vi "Write eLogLvl.vi"(8 "error in (no error)":errorcluster, 10 "eLogLvl":T1, 11 "Config in":refnum<class "Config.lvclass">) -> (0 "error out":errorcluster, 3 "Config out":refnum<class "Config.lvclass">)   [LabVIEW 2017, in "Framework.lvlib" / "Config.lvclass"]
uses:
  Config.lvclass
  Typedefs/eLogLvl.ctl
  Config.lvclass/Config.ctl
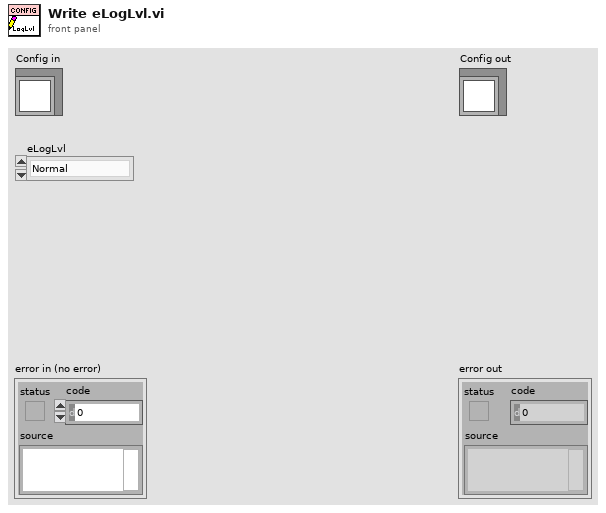
[diagram p1: front panel]
types:
  T1 = typedef "Framework.lvlib/Config.lvclass/eLogLvl.ctl" = enum16{"Normal", "Verbose", "None"}
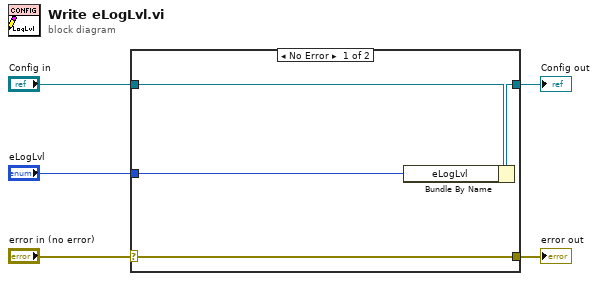
[diagram p0: block diagram]
diagram:
  n1 = case shown="No Error" "error in (no error)" {
    selector: "error in (no error)" -> [w9 w10]
    tunnel: [w9 w10] -> w4
    tunnel: [w7 w11] -> w2
    tunnel: "Config in" -> [w8 w11]
    tunnel: "eLogLvl" -> [w6 _]
    frame No Error {
      n2 = Bundle By Name(cluster=w8, "eLogLvl"=w6) -> (w7:refnum<class "Config.lvclass">)
    }
    frame Error {
    }
  }
  "error out" <- w4
  "Config out" <- w2
